vi "校验license.vi"(8 "error in (no error)":errorcluster caption="错误输入（无错误）", 11 "license":string) -> (0 "error out":errorcluster caption="错误输出", 3 "license正确":bool, 4 "授权类型":i32, 5 "T":u32)   [LabVIEW 2014]
uses:
  <userlib>/_OpenG.lib/md5/md5.llb/MD5 Message Digest (Hexadecimal String)__ogtk.vi
panel:
  out "数组":string[](array[string])
  out "子字符串":string
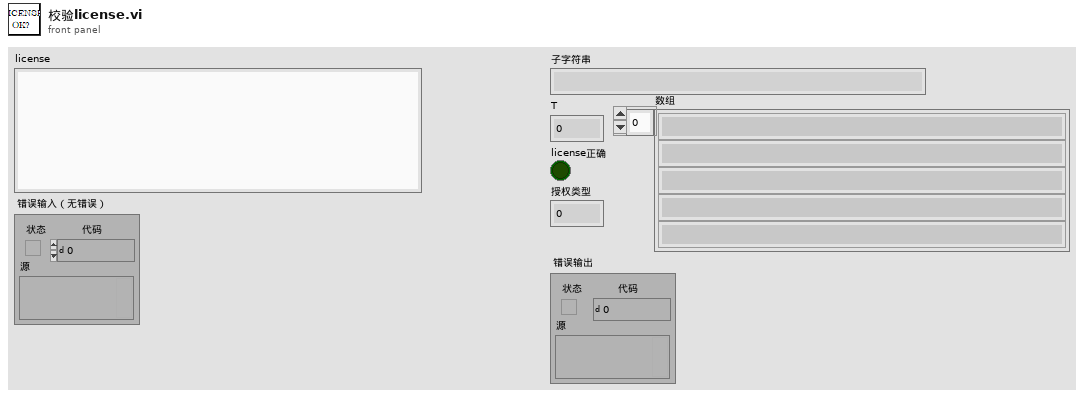
[diagram p1: front panel]
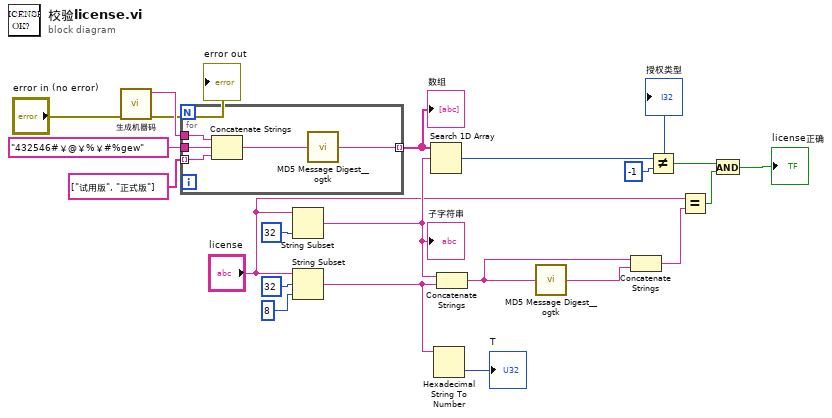
[diagram p0: block diagram]
diagram:
  n1 = call "生成机器码.vi"("error in (no error)"="error in (no error)") -> ("error out"=→"error out":errorcluster, "机器码"=w21:string)  [unwired: 9 in]
  n2 = for {
    tunnel: w21 -> [w24]
    tunnel: string[] ["试用版", "正式版"] ("字符串[]") -> [w22] mode=indexing
    tunnel: "432546#￥@￥%￥#%gew" -> [w23]
    tunnel: [w25] -> w14 mode=indexing
    n3 = Concatenate Strings(w24, w23, w22) -> (w26:string)
    n4 = call-poly <userlib>:"MD5 Message Digest__ogtk.vi"("Message"=w26) -> ("MD5 Message Digest"=w25:string)
  }
  "数组" <- w14
  n5 = String Subset(string="license", length (rest)=32 ("长度（剩余）")) -> (substring=w11:string)  [unwired: 1 in]
  "子字符串" <- w11
  n6 = String Subset(string="license", offset (0)=32 ("偏移量(0)"), length (rest)=8 ("长度（剩余）")) -> (substring=w10:string)
  n7 = Search 1D Array(1D array=w14, element=w11) -> (index of element=w13:i32)  [unwired: 1 in]
  "授权类型" <- w13
  n8 = Hexadecimal String To Number(string=w10) -> (number=→"T":u32)  [unwired: 2 in, 1 out]
  n9 = Concatenate Strings(w11, w10) -> (w7:string)
  n10 = call-poly <userlib>:"MD5 Message Digest__ogtk.vi"("Message"=w7) -> ("MD5 Message Digest"=w8:string)
  n11 = Concatenate Strings(w7, w8) -> (w6:string)
  n12 = Not Equal?(x=w13, y=-1) -> (x != y?=w5:bool)
  n13 = Equal?(x="license", y=w6) -> (x = y?=w4:bool)
  n14 = And(x=w5, y=w4) -> (x .and. y?=→"license正确":bool)
